vi "AFG3352X.add services for add channels.vi"(0 "i ref in":refnum<vi>, 3 "ms timeout (10000)":i32=10000, 5 "error in (no error)":errorcluster) -> (14 "i ref out":refnum<vi>, 17 "timed out":bool, 19 "error out":errorcluster)   [LabVIEW 2014, in "AFG3352X.lvlib"]
doc: "Declares the required DIM services."
uses:
  AFG3352X.lvlib
  CSlibraries-extern/DimLVEvent/LVDimInterface/LVDimInterface.lvlib
  CSCore/CSSystem/CSSystemLib/CSSystemLib.lvlib
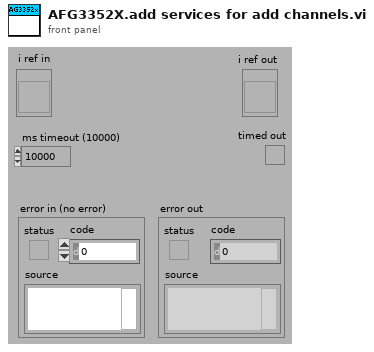
[diagram p1: front panel]
types:
  T1 = typedef "AFG3352X.lvlib/AFG3352X.i attribute.ctl" = cluster{"Act2ndValues":cluster{"frequency":dbl, "amplitude":dbl, "phase":dbl, "DCOffset":dbl, "waveformType":T2, "enableOutput":bool, "trigger":i16[], "serviceIDs":cluster{"frequencyID":i32, "amplitudeID":i32, "phaseID":i32, "DCOffsetID":i32, "waveformTypeID":i32, "enableOutputID":i32, "triggerID":i32}, "waveform":cluster{"data":waveform(dbl), "gain":dbl, "offset":dbl, "repetitionRate":dbl, "sampleRate":dbl}}, "Nom2ndValues":cluster{"frequency":dbl, "amplitude":dbl, "phase":dbl, "DCOffset":dbl, "waveformType":T2, "enableOutput":bool, "trigger":i16[], "serviceIDs":cluster{"frequencyID":i32, "amplitudeID":i32, "phaseID":i32, "DCOffsetID":i32, "waveformTypeID":i32, "enableOutputID":i32, "triggerID":i32}, "waveform":cluster{"data":waveform(dbl), "gain":dbl, "offset":dbl, "repetitionRate":dbl, "sampleRate":dbl}}, "DefaultChannel":i32, "ActAddValues":cluster{"Mode1":u16, "serviceIDs":cluster{"Mode1ID":i32, "Mode2ID":i32, "Burst1ID":i32, "Burst2ID":i32}, "Mode2":u16, "Burst1":i32, "Burst2":i32}, "NomAddValues":cluster{"Mode1":u16, "serviceIDs":cluster{"Mode1ID":i32, "Mode2ID":i32, "Burst1ID":i32, "Burst2ID":i32}, "Mode2 2":u16, "Burst1":i32, "Burst2":i32}, "enableBurstMode":bool}
  T2 = typedef "AFGBase.lvlib/AFGBase.waveformType.ctl" = enum16{"sine", "square", "ramp", "pulse", "noise", "DC", "arbitrary", "triangle", "ramp_up", "ramp_down", "amplitude modulation"}
  T3 = cluster{"my_serviceID":i32, "my_serviceID":i32, "my_serviceID":i32, "my_serviceID":i32}
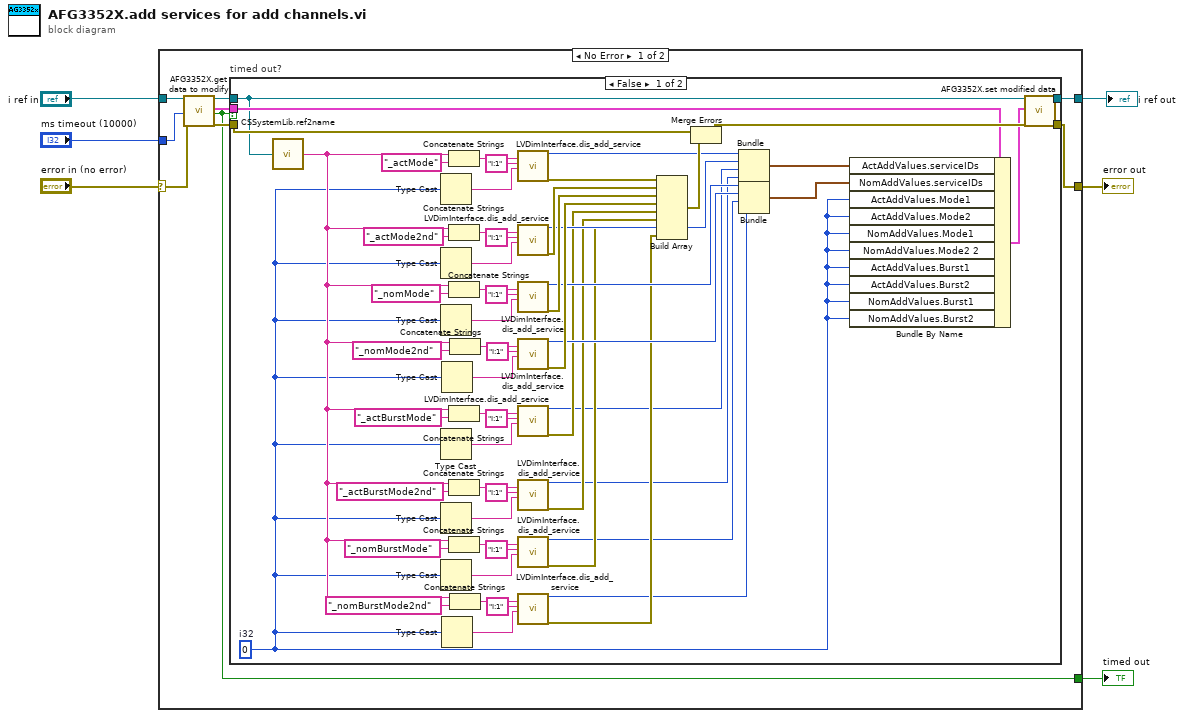
[diagram p0: block diagram]
diagram:
  n1 = case shown="No Error" "error in (no error)" {
    selector: "error in (no error)" -> [w13 w79]
    tunnel: [w9 w79] -> w5
    tunnel: "i ref in" -> [w15 w78]
    tunnel: [w11 w78] -> w1
    tunnel: "ms timeout (10000)" -> [w14 _]
    tunnel: [w8 _] -> w3
    frame No Error {
      n2 = call "AFG3352X.get data to modify.vi"("i ref in"=w15, "ms timeout (10000)"=w14, "error in (no error)"=w13) -> ("i ref out"=w12:refnum<vi>, "i attribute"=w7:T1, "timed out"=w8:bool, "error out"=w10:errorcluster)  [unwired: 13 in]
      n3 = case "timed out?" shown="False" w8 {
        tunnel: w12 -> [w46 w77]
        tunnel: [w75 w77] -> w11
        tunnel: w10 -> [w53 w76]
        tunnel: [w74 w76] -> w9
        tunnel: w7 -> [w50 _]
        frame False {
          w16 = 0  # i32
          n4 = call "CSSystemLib.ref2name.vi"("obj refnum"=w46) -> ("name"=w25:string)
          n5 = Type Cast(x=w16) -> (*(type *) &x=w70:string)  [unwired: 1 in]
          n6 = Type Cast(x=w16) -> (*(type *) &x=w69:string)  [unwired: 1 in]
          n7 = Type Cast(x=w16) -> (*(type *) &x=w62:string)  [unwired: 1 in]
          n8 = Type Cast(x=w16) -> (*(type *) &x=w38:string)  [unwired: 1 in]
          n9 = Type Cast(x=w16) -> (*(type *) &x=w37:string)  [unwired: 1 in]
          n10 = Type Cast(x=w16) -> (*(type *) &x=w30:string)  [unwired: 1 in]
          n11 = Type Cast(x=w16) -> (*(type *) &x=w58:string)  [unwired: 1 in]
          n12 = Type Cast(x=w16) -> (*(type *) &x=w26:string)  [unwired: 1 in]
          n13 = Concatenate Strings(w25, "_actMode" ("string")) -> (w73:string)
          n14 = Concatenate Strings(w25, "_actMode2nd" ("string")) -> (w66:string)
          n15 = Concatenate Strings(w25, "_nomMode" ("string")) -> (w65:string)
          n16 = Concatenate Strings(w25, "_actBurstMode" ("string")) -> (w41:string)
          n17 = Concatenate Strings(w25, "_actBurstMode2nd" ("string")) -> (w34:string)
          n18 = Concatenate Strings(w25, "_nomBurstMode" ("string")) -> (w33:string)
          n19 = Concatenate Strings(w25, "_nomMode2nd" ("string")) -> (w61:string)
          n20 = Concatenate Strings(w25, "_nomBurstMode2nd" ("string")) -> (w29:string)
          n21 = call "LVDimInterface.dis_add_service.vi"("serviceName"=w73, "typeDescriptor"="I:1", "data"=w70) -> ("my_serviceID"=w49:i32, "error out"=w57:errorcluster)  [unwired: 15 in]
          n22 = call "LVDimInterface.dis_add_service.vi"("serviceName"=w66, "typeDescriptor"="I:1", "data"=w69) -> ("my_serviceID"=w48:i32, "error out"=w56:errorcluster)  [unwired: 15 in]
          n23 = call "LVDimInterface.dis_add_service.vi"("serviceName"=w65, "typeDescriptor"="I:1", "data"=w62) -> ("my_serviceID"=w45:i32, "error out"=w55:errorcluster)  [unwired: 15 in]
          n24 = call "LVDimInterface.dis_add_service.vi"("serviceName"=w61, "typeDescriptor"="I:1", "data"=w58) -> ("my_serviceID"=w44:i32, "error out"=w54:errorcluster)  [unwired: 15 in]
          n25 = call "LVDimInterface.dis_add_service.vi"("serviceName"=w41, "typeDescriptor"="I:1", "data"=w38) -> ("my_serviceID"=w20:i32, "error out"=w24:errorcluster)  [unwired: 15 in]
          n26 = call "LVDimInterface.dis_add_service.vi"("serviceName"=w34, "typeDescriptor"="I:1", "data"=w37) -> ("my_serviceID"=w19:i32, "error out"=w23:errorcluster)  [unwired: 15 in]
          n27 = call "LVDimInterface.dis_add_service.vi"("serviceName"=w33, "typeDescriptor"="I:1", "data"=w30) -> ("my_serviceID"=w18:i32, "error out"=w22:errorcluster)  [unwired: 15 in]
          n28 = call "LVDimInterface.dis_add_service.vi"("serviceName"=w29, "typeDescriptor"="I:1", "data"=w26) -> ("my_serviceID"=w17:i32, "error out"=w21:errorcluster)  [unwired: 15 in]
          n29 = Build Array(w57, w56, w55, w54, w24, w23, w22, w21) -> (w52:errorcluster[])
          n30 = Merge Errors(w53, w52) -> (w51:errorcluster)
          n31 = Bundle("my_serviceID"=w49, "my_serviceID"=w48, "my_serviceID"=w20, "my_serviceID"=w19) -> (w43:T3)  [unwired: 1 in]
          n32 = Bundle("my_serviceID"=w45, "my_serviceID"=w44, "my_serviceID"=w18, "my_serviceID"=w17) -> (w42:T3)  [unwired: 1 in]
          n33 = Bundle By Name(cluster=w50, "ActAddValues.serviceIDs"=w43, "NomAddValues.serviceIDs"=w42, "ActAddValues.Mode1"=w16, "ActAddValues.Mode2"=w16, "NomAddValues.Mode1"=w16, "NomAddValues.Mode2 2"=w16, "ActAddValues.Burst1"=w16, "ActAddValues.Burst2"=w16, "NomAddValues.Burst1"=w16, "NomAddValues.Burst2"=w16) -> (w47:T1)
          n34 = call "AFG3352X.set modified data.vi"("i ref in"=w46, "i attribute"=w47, "error in (no error)"=w51) -> ("i ref out"=w75:refnum<vi>, "error out"=w74:errorcluster)  [unwired: 15 in]
        }
        frame True {
        }
      }
    }
    frame Error {
    }
  }
  "error out" <- w5
  "timed out" <- w3
  "i ref out" <- w1
